vi "Add Minor Frames.vi"(8 "error in (no error)":errorcluster, 10 "Minor Frames":refnum<class "Minor Frame.lvclass">[](array[class]), 11 "Major Frame in":refnum<class "Major Frame.lvclass">) -> (0 "error out":errorcluster, 3 "Major Frame out":refnum<class "Major Frame.lvclass">)   [LabVIEW 2020, in "BCI-1553 API.lvlib" / "Major Frame.lvclass"]
doc: "Adds Minor Frames to the Major Frame. If two Minor Frames have conflicting IDs, the latest Minor Frame will take priority and overwrite the previous one.\n\nNote: This method does not modify the Schedule."
uses:
  Major Frame.lvclass
  Minor Frame/Minor Frame.lvclass
  Major Frame.lvclass/Major Frame.ctl
  Dependencies/Registry/Registry.lvclass/Registry.ctl
  Dependencies/Registry/Add Entry.vi
  Dependencies/Registry/Registry.lvclass
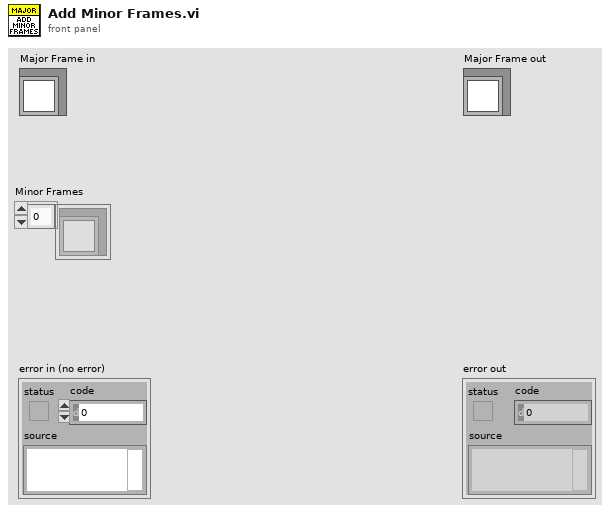
[diagram p1: front panel]
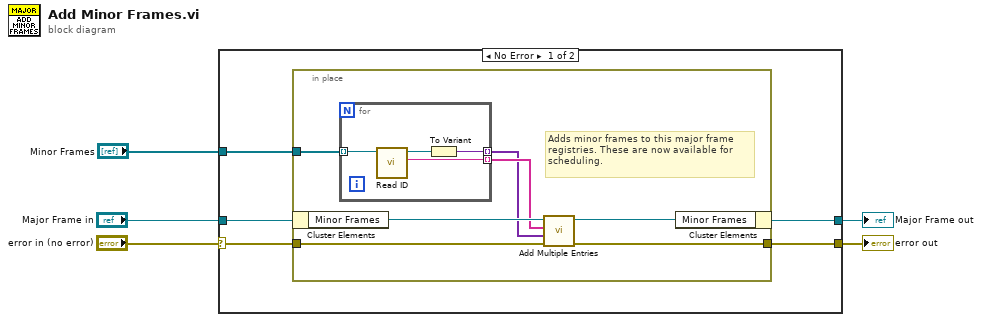
[diagram p0: block diagram]
diagram:
  n1 = case shown="No Error" "error in (no error)" {
    selector: "error in (no error)" -> [w7 w23]
    tunnel: [w8 w23] -> w4
    tunnel: [w9 w22] -> w2
    tunnel: "Major Frame in" -> [w10 w22]
    tunnel: "Minor Frames" -> [w6 _]
    frame No Error {
      n2 = in-place {
        in-place-border: [w15] -> w8
        in-place-border: w7 -> [w14]
        in-place-border: w6 -> [w13]
        # "Adds minor frames to this major frame\nregistries. These are now available for\nscheduling."
        n3 = in-place-cluster #1(w10) -> ("Minor Frames"=w17:refnum<class "Registry.lvclass">)
        n4 = for {
          tunnel: w13 -> [w21] mode=indexing
          tunnel: [w20] -> w12 mode=indexing
          tunnel: [w18] -> w11 mode=indexing
          n5 = call-dynamic "Read ID.vi"("Minor Frame in"=w21) -> ("ID"=w20:string, "Minor Frame out"=w19:refnum<class "Minor Frame.lvclass">)  [unwired: 8 in, 1 out]
          n6 = To Variant(anything=w19) -> (Variant=w18:variant)
        }
        n7 = call "Add Multiple Entries.vi"("error in (no error)"=w14, "Values"=w11, "Keys"=w12, "Registry in"=w17) -> ("error out"=w15:errorcluster, "Registry out"=w16:refnum<class "Registry.lvclass">)  [unwired: 5 in, 1 out]
        n8 = in-place-cluster #1("Minor Frames"=w16) -> (w9:refnum<class "Major Frame.lvclass">)
      }
    }
    frame Error {
    }
  }
  "error out" <- w4
  "Major Frame out" <- w2
